vi "FT_Get_Com_Port.vi"(8 "error in (no error)":errorcluster, 11 "Handle In":u64) -> (0 "error out":errorcluster, 1 "FT_Status":u32(ring) items=["FT_OK", "FT_INVALID_HANDLE", "FT_DEVICE_NOT_FOUND", "FT_DEVICE_NOT_OPENED", "FT_IO_ERROR", "FT_INSUFFICIENT_RESOURCES", "FT_INVALID_PARAMETER", "FT_INVALID_BAUD_RATE", "FT_DEVICE_NOT_OPENED_FOR_ERASE", "FT_DEVICE_NOT_OPENED_FOR_WRITE", "FT_FAILED_TO_WRITE_DEVICE", "FT_EEPROM_READ_FAILED", "FT_EEPROM_WRITE_FAILED", "FT_EEPROM_ERASE_FAILED", "FT_EEPROM_NOT_PRESENT", "FT_EEPROM_NOT_PROGRAMMED", "FT_INVALID_ARGS", "FT_NOT_SUPPORTED", "FT_OTHER_ERROR"], 2 "ComPortNumber":i32, 3 "Handle Out":u64)   [LabVIEW 2020]
uses:
  FTD2XX.dll
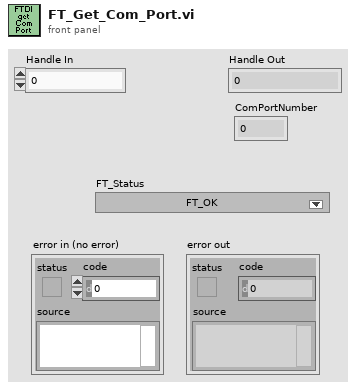
[diagram p1: front panel]
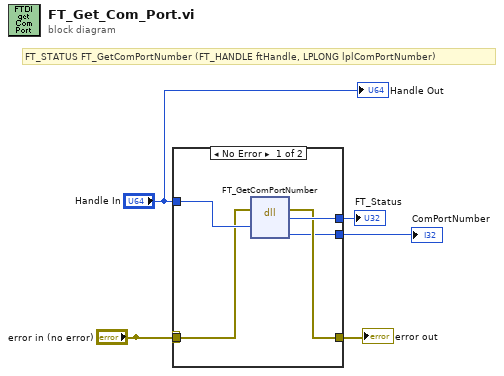
[diagram p0: block diagram]
diagram:
  # "FT_STATUS FT_GetComPortNumber (FT_HANDLE ftHandle, LPLONG lplComPortNumber)"
  n1 = case shown="No Error" "error in (no error)" {
    selector: "error in (no error)" -> [_ w11]
    tunnel: "Handle In" -> [w10 _]
    tunnel: [w9 _] -> w5
    tunnel: [w7 w11] -> w4
    tunnel: "error in (no error)" -> [w8 _]
    tunnel: [w6 _] -> w1
    frame No Error {
      n2 = dll-call lib="FTD2XX.dll" fn="FT_GetComPortNumber"(error in=w8, "Handle"=w10) -> (error out=w7:errorcluster, "FT_Status"=w9:u32, "ComPortNumber"=w6:i32)  [unwired: 4 in, 1 out]
    }
    frame Error {
    }
  }
  "FT_Status" <- w5
  "error out" <- w4
  "ComPortNumber" <- w1
  "Handle Out" <- "Handle In"
